vi "Functional Imaging-Remove specified POI.vi"(8 "error in (no error)":errorcluster, 10 "Index of POI to delete":i16) -> (0 "error out":errorcluster, 1 "Updated [POI#]":T1 {"ROI number" min=1 format="ROI %.0f"})   [LabVIEW 2017]
uses:
  Typedefs/ROI selector array-ROI vis.ctl
  xcontrol/Interface VIs/Interface typedefs/Interface-ROI selection cluster.ctl
  Typedefs/ROI ID Enum.ctl
  Global variables/gl_Functional Imaging-Global variables.vi
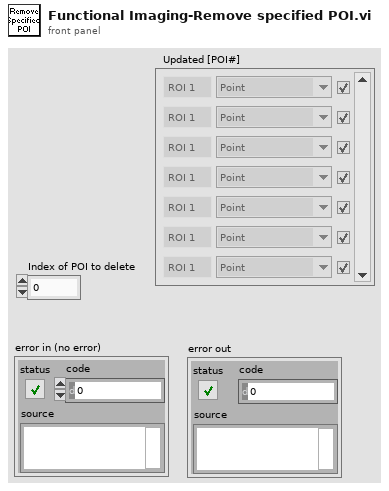
[diagram p1: front panel]
types:
  T1 = typedef "ROI selector array-ROI vis.ctl" = T2[]
  T2 = typedef "Interface-ROI selection cluster.ctl" = cluster{"ROI number":i32, "ROI ID":T3, "Visibility":bool}
  T3 = typedef "ROI ID Enum.ctl" = enum16{"Point", "MiniScan", "Comp. MiniScan", "Rectangle", "Comp. volume", "Arb. plane point"}
  T4 = typedef "Functional Imging UI Refs.ctl" = cluster{"Menu ref":refnum<k9>, "Image control":refnum<vi>, "VI ref":refnum<vi>, "XGrapher":refnum<vi>, "Smoothing":refnum<vi>, "POI Averaging":refnum<vi>, "Normalize":refnum<vi>, "POI data points in each trial":refnum<vi>, "Channel":refnum<vi>, "Experiment data folder path":refnum<vi>, "[ROI vis]":refnum<vi>, "[Groups] visbl":T5, "Group Name":refnum<vi>, "POI index":refnum<vi>, "Trial No.":refnum<vi>, "Intensity Zoom":refnum<vi>, "Trial Cursor Enabled":refnum<vi>, "Number of Trials (ind 1)":refnum<vi>, "Number of Trials (ind 2)":refnum<vi>, "MiniScans Available":refnum<vi>, "POI Available":refnum<vi>, "Defer graph updates":refnum<vi>, "Waveform selector":refnum<vi>, "#of selected POI":refnum<vi>, "#of selected MiniScans":refnum<vi>, "#of selected groups":refnum<vi>, "Max Z-Projection":refnum<vi>, "Z-Plane Selector":refnum<vi>, "Index of miniscan point to visualise":refnum<vi>, "ROI vis. mode":refnum<vi>, "Total # of points":refnum<vi>, "Index of group clicked on":refnum<vi>, "Pane 1":refnum<vi>, "Pane 2":refnum<vi>, "Pane 3":refnum<vi>, "Pane 4":refnum<vi>, "Pane 5":refnum<vi>, "Pane 6":refnum<vi>, "Deselect all ROI":refnum<vi>, "Deselect all groups":refnum<vi>}
  T5 = typedef "Groups array referecne.ctl" = refnum<vi>
  T6 = typedef "ROI selector array.ctl" = T2[]
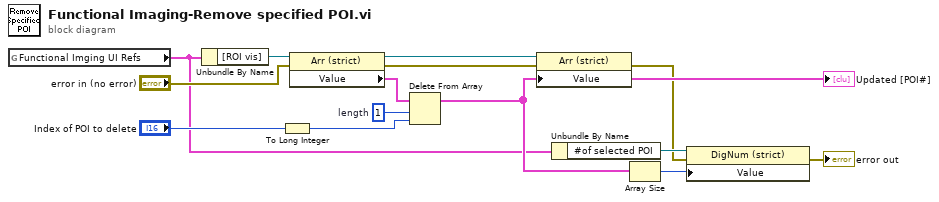
[diagram p0: block diagram]
diagram:
  w8 = 1  # length
  n1 = global read "gl_Functional Imaging-Global variables.vi" "Functional Imging UI Refs"() -> (w1:T4)
  n2 = Unbundle By Name(w1) -> ("[ROI vis]"=w13:refnum<vi>)
  n3 = To Long Integer(number="Index of POI to delete") -> (32bit integer=w3:i32)
  n4 = property on="Property Node" class="Arr (strict)"(reference=w13, error in="error in (no error)") -> (reference out=w14:refnum<vi>, error out=w11:errorcluster, "Value"=w9:T6)
  n5 = Delete From Array "Delete From Array"(array=w9, length=w8, index=w3) -> (array with subset deleted=w5:T6)  [unwired: 1 out]
  "Updated [POI#]" <- w5
  n6 = property on="Property Node" class="Arr (strict)"(reference=w14, error in=w11, "Value"=w5) -> (error out=w4:errorcluster)  [unwired: 1 out]
  n7 = Unbundle By Name(w1) -> ("#of selected POI"=w7:refnum<vi>)
  n8 = Array Size(array=w5) -> (size(s)=w6:i32)
  n9 = property on="Property Node" class="DigNum (strict)"(reference=w7, error in=w4, "Value"=w6) -> (error out=→"error out":errorcluster)  [unwired: 1 out]
